vi "keithly set-up.vi"(8 "error in":errorcluster, 10 "ConfigOpt":i16(ring)=1 items=["SAV0", "SAV1", "SAV2", "SAV3", "SAV4", "SAV5", "SAV6", "SAV7", "SAV8", "SAV9", "RST", "Preset"], 11 "GPIB Address":string="27") -> (0 "error out":errorcluster, 2 "Instrument ID String":string="KEITHLEY INSTRUMENTS INC.,MODEL 6517B,1253950,A06/700x \nKEITHLEY INSTRUMENTS INC.,MODEL 6517B,1253950,A06/700x \nKEITHLEY INSTRUMENTS INC.,MODEL 6517B,1253950,A06/700x \nKEITHLEY INSTRUMENTS INC.,MODEL 6517B,1253950,A06/700x \nKEITHLEY INSTRUMENTS INC.,MODEL 6517B,1253950,A06/700x \nKEITHLEY INSTRUMENTS INC.,MODEL 6517B,1253950,A06/700x ", 3 "GPIB Address out":string="27")   [LabVIEW 2024]
doc: "VI intializes connection to Keithley 6517 picoampmeter (K6517) to read photodiode currents for reflectivity test station.\n\nK6517 must be connected to to PC via GPIB."
panel:
  # "Start Keithley 6517 Electrometer"
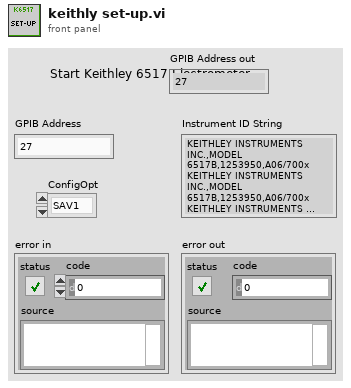
[diagram p1: front panel]
types:
  T1 = cluster{"error":bool, "code":i32, "source":string}
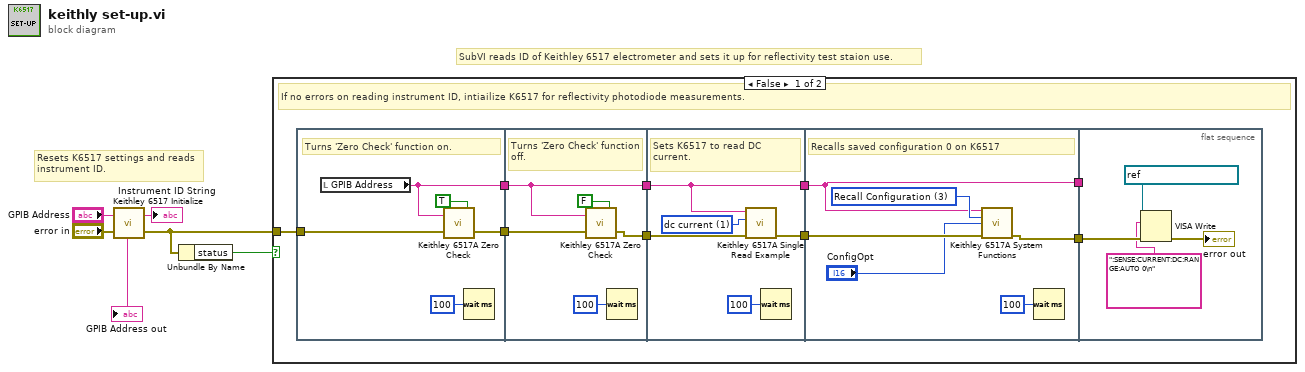
[diagram p0: block diagram]
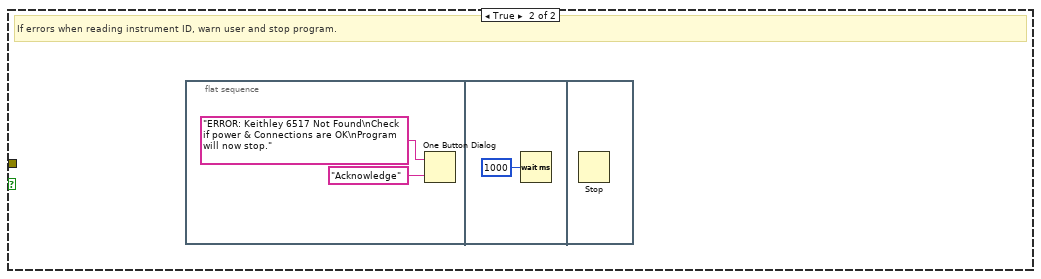
[diagram p2: hidden frame]
diagram:
  # "Resets K6517 settings and reads\ninstrument ID."
  # "SubVI reads ID of Keithley 6517 electrometer and sets it up for reflectivity test staion use."
  n1 = call "Keithley 6517 Initialize.vi"("error in (no error)"="error in", "GPIB Address"="GPIB Address") -> ("error out copy"=w5:errorcluster, "Instrument ID String"=→"Instrument ID String":string)
  n2 = Unbundle By Name(w5) -> ("status"=w4:bool)
  n3 = case shown="False" w4 {
    tunnel: w5 -> [w11 _]
    frame False {
      # "If no errors on reading instrument ID, intiailize K6517 for reflectivity photodiode measurements."
      n4 = flat-sequence {
        tunnel: w11 -> [w18]
        tunnel: [w17] -> w14
        tunnel: [w16] -> w10
        tunnel: w14 -> [w23]
        tunnel: [w22] -> w13
        tunnel: w10 -> [w21]
        tunnel: [w21] -> w9
        tunnel: w13 -> [w28]
        tunnel: [w27] -> w12
        tunnel: w9 -> [w26]
        tunnel: [w26] -> w8
        tunnel: w12 -> [w34]
        tunnel: w8 -> [w30]
        tunnel: [w31] -> w7
        tunnel: [w30] -> w6
        tunnel: w7 -> [w39]
        tunnel: w6 -> [_]
        frame #0 {
          # "Turns 'Zero Check' function on."
          n5 = local read "GPIB Address"() -> (w16:string)
          n6 = call "Keithley 6517A Zero Check.vi"("Zero Check"=TRUE, "error in"=w18, "GPIB address"=w16) -> ("error out"=w17:T1)
          n7 = Wait (ms)(milliseconds to wait=u32 100) -> ()  [unwired: 1 out]
        }
        frame #1 {
          # "Turns 'Zero Check' function off."
          n8 = call "Keithley 6517A Zero Check.vi"("Zero Check"=FALSE, "error in"=w23, "GPIB address"=w21) -> ("error out"=w22:T1)
          n9 = Wait (ms)(milliseconds to wait=u32 100) -> ()  [unwired: 1 out]
        }
        frame #2 {
          w25 = u16 1 items=["dc voltage", "dc current", "resistance", "charge"] ("function (Vdc:0)")
          # "Sets K6517 to read DC current."
          n10 = call "Keithley 6517A Single Read Example.vi"("GPIB address"=w26, "function (Vdc:0)"=w25, "error in"=w28) -> ("error out"=w27:T1)  [unwired: 2 in, 4 out]
          n11 = Wait (ms)(milliseconds to wait=u32 100) -> ()  [unwired: 1 out]
        }
        frame #3 {
          w33 = u16 3 items=["Reset Reading Number", "Reset Relative Timestamp", "Save Configuration", "Recall Configuration", "Set Power-On State", "Line-Sync Controls", "Set Time and Date", "Select Timestamp Type", "External Temperature Control", "A/D Hardware Limit Control", "Humidity Reading Control"] ("System Functions")
          # "Recalls saved configuration 0 on K6517"
          n12 = call "Keithley 6517A System Functions.vi"("GPIB address"=w30, "System Functions"=w33, "Save, Recall, or Power-on Selection"="ConfigOpt", "error in"=w34) -> ("error out"=w31:T1)  [unwired: 11 in]
          n13 = Wait (ms)(milliseconds to wait=u32 100) -> ()  [unwired: 1 out]
        }
        frame #4 {
          n14 = VISA Write(VISA resource name=refnum<visa-resource-name> "GPIB0::27::INSTR", write buffer=":SENSE:CURRENT:DC:RANGE:AUTO 0\n", error in (no error)=w39) -> (error out=→"error out":errorcluster)  [unwired: 2 out]
        }
      }
    }
    frame True {
      # "If errors when reading instrument ID, warn user and stop program."
      n15 = flat-sequence {
        frame #0 {
          n16 = One Button Dialog(message="ERROR: Keithley 6517 Not Found\nCheck if power & Connections are OK\nProgram will now stop.", button name ("OK")="Acknowledge") -> ()  [unwired: 1 out]
        }
        frame #1 {
          n17 = Wait (ms)(milliseconds to wait=u32 1000) -> ()  [unwired: 1 out]
        }
        frame #2 {
          n18 = Stop() -> ()  [unwired: 1 in]
        }
      }
    }
  }
  "GPIB Address out" <- "GPIB Address"
